vi "access table insert sqlite.vi"(8 "error in (no error)":errorcluster, 10 "table":string, 11 "路径":path) -> (0 "错误输出":errorcluster, 3 "条数":i32)   [LabVIEW 2016]
uses:
  <vilib>/addons/database/Connection.llb/DB Tools Open Connec (String).vi
  <vilib>/addons/database/NI_Database_API.lvlib
  SQLite/SQLite Lib.lvlib
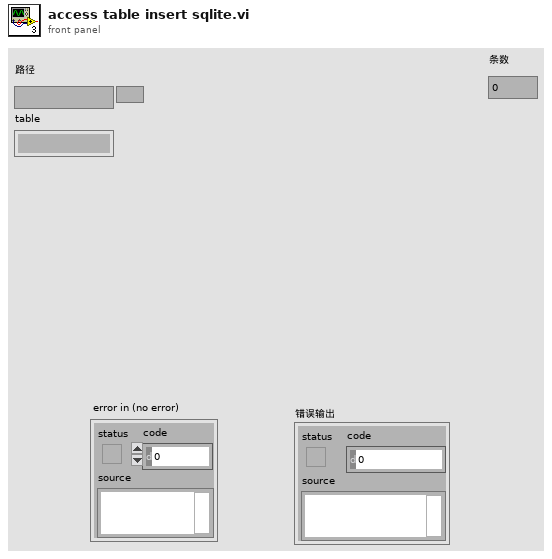
[diagram p1: front panel]
types:
  T1 = cluster{"columns外部输入":bool, "columns input":string[]}
  T2 = typedef "NI_Database_API.lvlib/Conn ObjectReference.ctl" = refnum<k1>
  T3 = typedef "NI_Database_API.lvlib/DB Tools DataTypes.ctl" = enum16{"String", "Long (I32)", "Single (SGL)", "Double (DBL)", "Date/Time", "Binary"}
  T4 = cluster{"name":string, "database data type":T3, "defined size":i32}[]
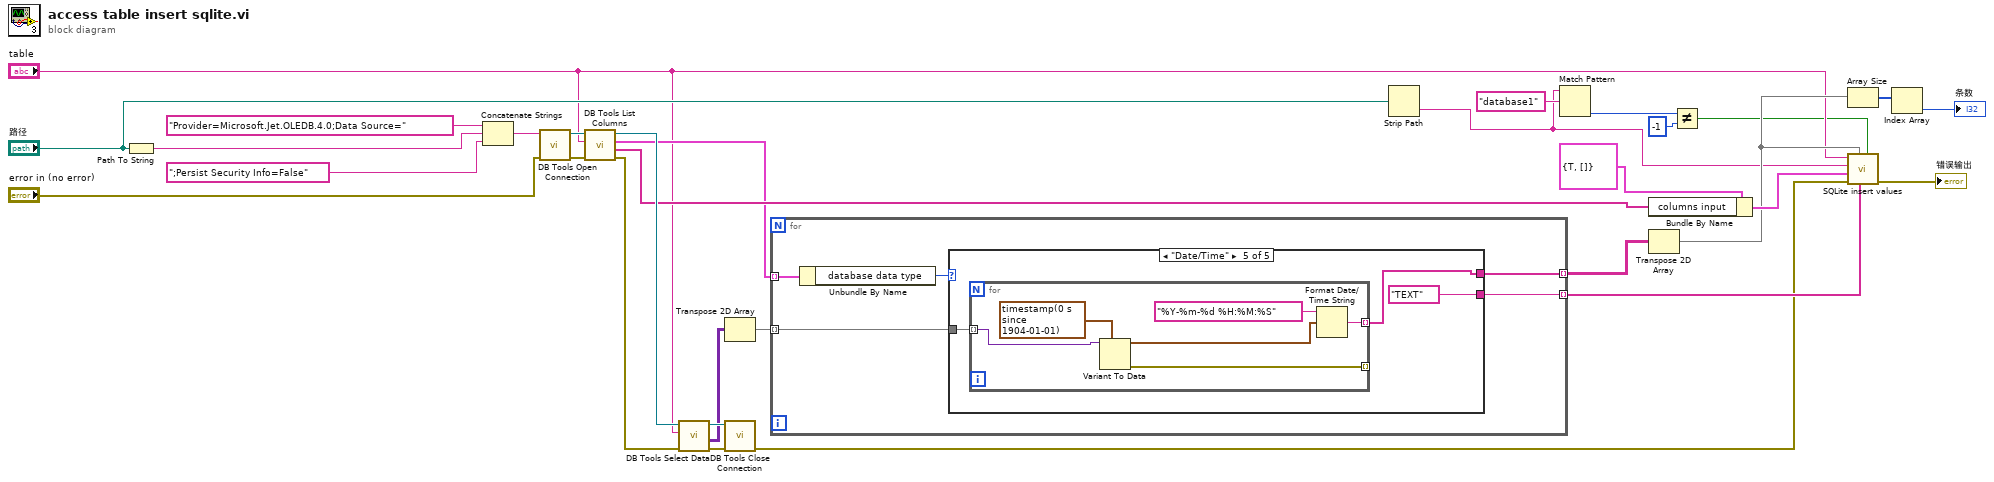
[diagram p0: block diagram]
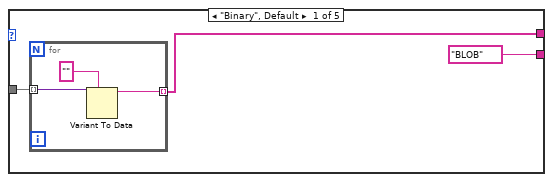
[diagram p2: hidden frame]
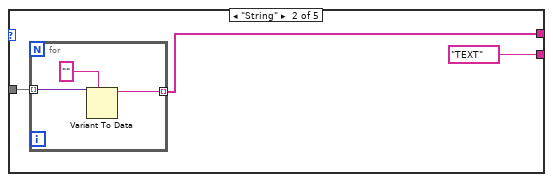
[diagram p3: hidden frame]
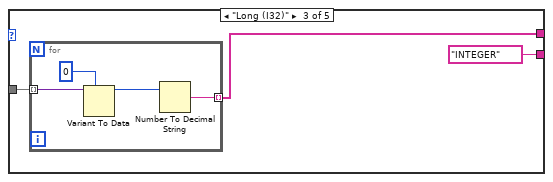
[diagram p4: hidden frame]
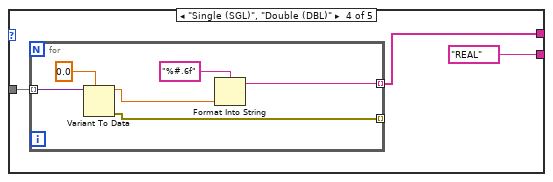
[diagram p5: hidden frame]
diagram:
  n1 = Path To String(path="路径") -> (string=w21:string)
  n2 = Concatenate Strings("Provider=Microsoft.Jet.OLEDB.4.0;Data Source=" ("condition"), w21, ";Persist Security Info=False" ("condition")) -> (w19:string)
  n3 = call-poly <vilib>:"DB Tools Open Connection.vi"("error in (no error)"="error in (no error)", "connection information"=w19) -> ("error out"=w27:errorcluster, "connection reference"=w31:T2)  [unwired: 6 in]
  n4 = call <vilib>:"DB Tools List Columns.vi"("error in (no error)"=w27, "table"="table", "connection reference"=w31) -> ("error out"=w26:errorcluster, "columns"=w23:string[], "column information"=w18:T4, "connection reference out"=w28:T2)  [unwired: 1 in]
  n5 = call <vilib>:"DB Tools Select Data.vi"("error in (no error)"=w26, "table"="table", "connection reference"=w28) -> ("error out"=w29:errorcluster, "data"=w16:variant[][], "connection reference out"=w30:T2)  [unwired: 3 in]
  n6 = Transpose 2D Array(2D array=w16) -> (transposed array=w15:variant[][])
  n7 = call <vilib>:"DB Tools Close Connection.vi"("error in (no error)"=w29, "connection reference"=w30) -> ("error out"=w13:errorcluster)  [unwired: 5 in]
  n8 = for {
    tunnel: w18 -> [w36] mode=indexing
    tunnel: [w34] -> w17 mode=indexing
    tunnel: w15 -> [w33] mode=indexing
    tunnel: [w32] -> w14 mode=indexing
    n9 = Unbundle By Name(w36) -> ("database data type"=w35:T3)
    n10 = case shown="\"Date/Time\"" w35 {
      tunnel: ["BLOB" ("组合框") "TEXT" ("组合框") "INTEGER" ("组合框") "REAL" ("组合框") "TEXT" ("组合框")] -> w34
      tunnel: w33 -> [w38 w44 w50 w57 w66]
      tunnel: [w37 w43 w49 w56 w65] -> w32
      frame "Binary", Default {
        n11 = for {
          tunnel: w38 -> [w41] mode=indexing
          tunnel: [w40] -> w37 mode=indexing
          n12 = Variant To Data(type="", Variant=w41) -> (data=w40:string)  [unwired: 1 in, 1 out]
        }
      }
      frame "String" {
        n13 = for {
          tunnel: w44 -> [w47] mode=indexing
          tunnel: [w46] -> w43 mode=indexing
          n14 = Variant To Data(type="", Variant=w47) -> (data=w46:string)  [unwired: 1 in, 1 out]
        }
      }
      frame "Long (I32)" {
        n15 = for {
          tunnel: w50 -> [w53] mode=indexing
          tunnel: [w52] -> w49 mode=indexing
          n16 = Variant To Data(type=0, Variant=w53) -> (data=w55:i32)  [unwired: 1 in, 1 out]
          n17 = Number To Decimal String(number=w55) -> (decimal integer string=w52:string)  [unwired: 1 in]
        }
      }
      frame "Single (SGL)", "Double (DBL)" {
        n18 = for {
          tunnel: w57 -> [w61] mode=indexing
          tunnel: [w60] -> w56 mode=indexing
          tunnel: [w59] -> _ mode=indexing
          n19 = Variant To Data(type=sgl 0.0, Variant=w61) -> (data=w63:sgl, error out=w59:errorcluster)  [unwired: 1 in]
          n20 = Format Into String(format string="%#.6f" ("格式字符串"), w63) -> (resulting string=w60:string)  [unwired: 2 in, 1 out]
        }
      }
      frame "Date/Time" {
        n21 = for {
          tunnel: w66 -> [w71] mode=indexing
          tunnel: [w69] -> w65 mode=indexing
          tunnel: [w68] -> _ mode=indexing
          n22 = Variant To Data(type=timestamp(0 s since 1904-01-01) ("时间标识"), Variant=w71) -> (data=w70:timestamp, error out=w68:errorcluster)  [unwired: 1 in]
          n23 = Format Date/Time String(time format string (%c)="%Y-%m-%d %H:%M:%S" ("时间格式字符串(%c)"), seconds (now)=w70) -> (date/time string=w69:string)  [unwired: 1 in]
        }
      }
    }
  }
  n24 = Strip Path(path="路径") -> (name=w1:string)  [unwired: 1 out]
  n25 = Match Pattern(string=w1, regular expression="database1" ("正则表达式")) -> (offset past match=w4:i32)  [unwired: 1 in, 3 out]
  n26 = Bundle By Name(cluster=T1 {"columns外部输入"=TRUE, "columns input"=[]} ("columns外部输入"), "columns input"=w23) -> (w24:T1)
  n27 = Transpose 2D Array(2D array=w14) -> (transposed array=w9:string[][])
  n28 = Not Equal?(x=w4, y=-1) -> (x != y?=w2:bool)
  n29 = Array Size(array=w9) -> (size(s)=w8:i32[])
  n30 = call "SQLite insert values.vi"("是否创建唯一键"=w2, "columns  INFO"=w17, "数组"=w9, "错误输入（无错误）"=w13, "columns外部输入"=w24, "database"=w1, "Tabe Name"="table") -> ("错误输出"=→"错误输出":errorcluster)  [unwired: 4 in]
  n31 = Index Array(array=w8) -> (element=→"条数":i32)  [unwired: 1 in]
